vi "Get Data SubBlocks.vi"(8 "错误输入":errorcluster, 10 "Offset In":i32, 11 "Gif data in":string) -> (0 "错误输出":errorcluster, 1 "Data Blocks":cluster{"Len":u8, "Gif data Out":string}[](array[cluster]), 2 "Offset Out":i32, 3 "Gif data out":string)   [LabVIEW 2011, in "Gif Image.lvclass"]
uses:
  Gif Image.lvclass
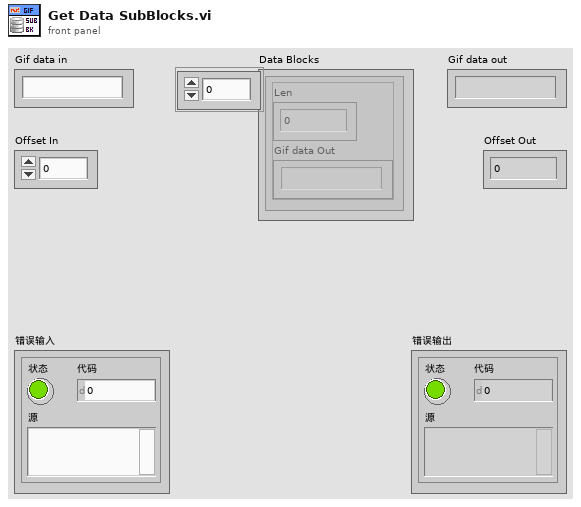
[diagram p1: front panel]
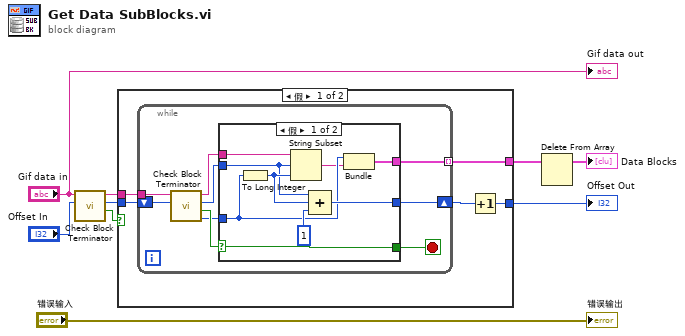
[diagram p0: block diagram]
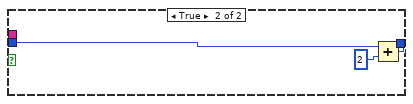
[diagram p3: hidden frame]
diagram:
  n1 = call "Check Block Terminator.vi"("Offset In"="Offset In", "Gif data in"="Gif data in") -> ("Block Terminator?"=w7:bool, "Offset Out"=w9:i32, "Gif data Out"=w6:string)  [unwired: 6 in, 1 out]
  n2 = case shown="假" w7 {
    tunnel: [w12 w36] -> w4
    tunnel: w6 -> [w14 _]
    tunnel: w9 -> [w11 w35]
    tunnel: [w10 _] -> w3
    frame False {
      n3 = while {
        shift-right: [w22] -> w13
        shift-left: w11 -> [w19]
        tunnel: w14 -> [w21]
        tunnel: [w15] -> w10 mode=indexing
        stop <- w23 stop-if-true
        n4 = call "Check Block Terminator.vi"("Offset In"=w19, "Gif data in"=w21) -> ("Len"=w16:u8, "Block Terminator?"=w17:bool, "Offset Out"=w18:i32, "Gif data Out"=w20:string)  [unwired: 6 in]
        n5 = case shown="假" w17 {
          selector: w17 -> [w32 w34]
          tunnel: [w32 w34] -> w23
          tunnel: [w29 w33] -> w22
          tunnel: w20 -> [w28 _]
          tunnel: w18 -> [w27 w33]
          tunnel: w16 -> [w26 _]
          tunnel: [w24 _] -> w15
          frame False {
            n6 = To Long Integer(number=w26) -> (32bit integer=w31:i32)
            n7 = String Subset(string=w28, offset (0)=w27, length (rest)=w31) -> (substring=w25:string)
            n8 = Compound Arithmetic op=ADD(w27, w31, 1 ("值")) -> (w29:i32)
            n9 = Bundle("Len"=w26, "Gif data Out"=w25) -> (w24:cluster{"Len":u8, "Gif data Out":string})  [unwired: 1 in]
          }
          frame True {
          }
        }
      }
      n10 = Increment(x=w13) -> (x+1=w12:i32)
    }
    frame True {
      n11 = Add(x=w35, y=2) -> (x+y=w36:i32)
    }
  }
  "Offset Out" <- w4
  n12 = Delete From Array(array=w3) -> (array with subset deleted=→"Data Blocks":cluster{"Len":u8, "Gif data Out":string}[])  [unwired: 2 in, 1 out]
  "Gif data out" <- "Gif data in"
  "错误输出" <- "错误输入"
